vi "Optimize Function.vi"(3 "output control":T1, 4 "data":variant, 5 "X":dbl[](array[numeric])) -> (0 "error out":errorcluster, 1 "gradient":dbl[](array[numeric]), 2 "f(X)":dbl)   [LabVIEW 2016]
doc: "Use this template VI as a starting point to create an objective function you want to pass to the Unconstrained Optimization VI."
uses:
  <vilib>/Utility/error.llb/Error Cluster From Error Code.vi
  <vilib>/ErrorRing/Error Ring.xnode
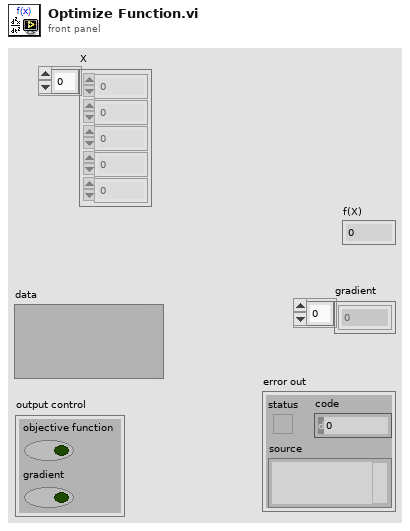
[diagram p1: front panel]
types:
  T1 = cluster{"objective function":bool, "gradient":bool}
  T2 = cluster{"c":dbl, "Intensity Graph":refnum<vi>, "animate?":bool}
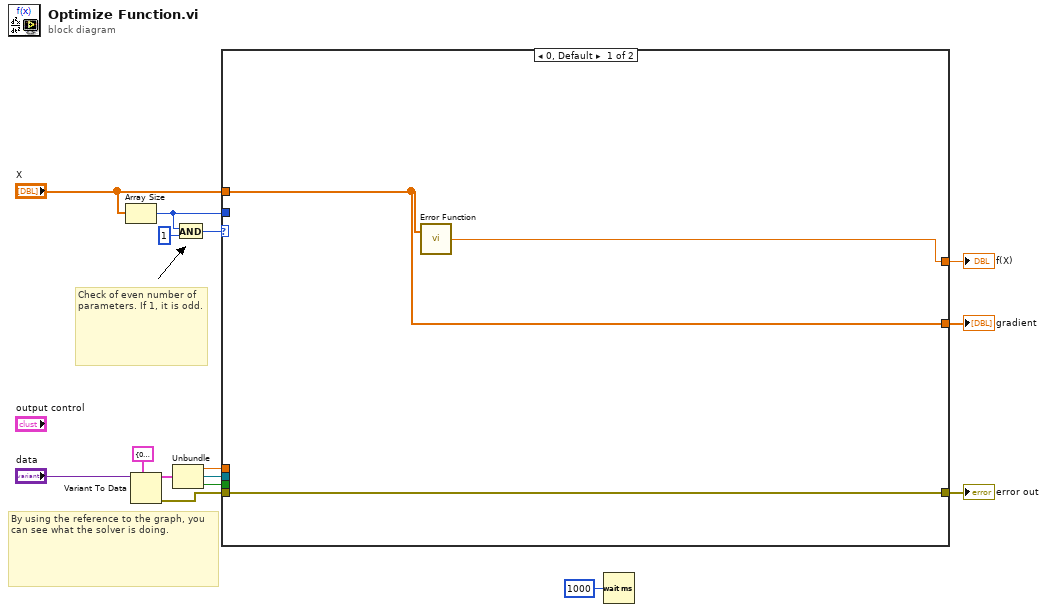
[diagram p0: block diagram]
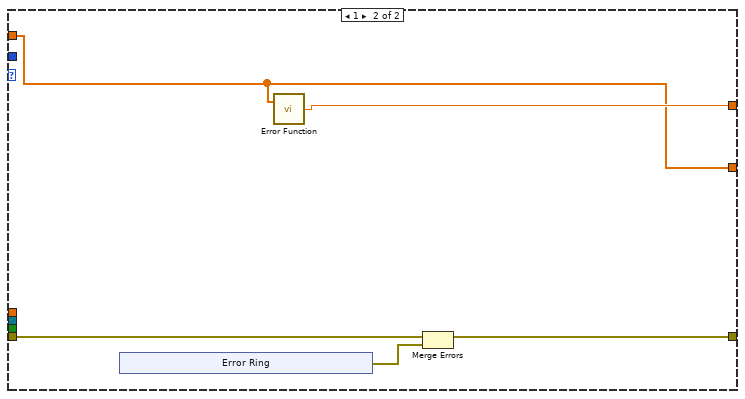
[diagram p2: hidden frame]
diagram:
  # "By using the reference to the graph, you can see what the solver is doing."
  # "Check of even number of parameters. If 1, it is odd."
  n1 = Array Size(array="X") -> (size(s)=w11:i32)
  n2 = Variant To Data(type=T2 {"c"=0.0, "Intensity Graph"=refnum, "animate?"=FALSE} ("output cluster"), Variant="data") -> (data=w9:T2, error out=w4:errorcluster)  [unwired: 1 in]
  n3 = Unbundle(w9) -> ("c"=w7:dbl, "Intensity Graph"=w6:refnum<vi>, "animate?"=w5:bool)
  n4 = And(x=w11, y=1) -> (x .and. y?=w14:i32)
  n5 = case shown="0, Default" w14 {
    tunnel: [w16 w22] -> w13
    tunnel: "X" -> [w17 w19]
    tunnel: w11 -> [_ _]
    tunnel: w7 -> [_ _]
    tunnel: w6 -> [_ _]
    tunnel: w5 -> [_ _]
    tunnel: w4 -> [w16 w23]
    tunnel: [w18 w20] -> w3
    tunnel: [w17 w19] -> w2
    frame 0, Default {
      n6 = call "Error Function.vi"("Array"=w17) -> ("Error"=w18:dbl)  [unwired: 1 in]
    }
    frame 1 {
      n7 = xnode "Error Ring"() -> ("error out"=w21:errorcluster)
      n8 = call "Error Function.vi"("Array"=w19) -> ("Error"=w20:dbl)  [unwired: 1 in]
      n9 = Merge Errors(w23, w21) -> (w22:errorcluster)
    }
  }
  "error out" <- w13
  "f(X)" <- w3
  "gradient" <- w2
  n10 = Wait (ms)(milliseconds to wait=u32 1000) -> ()  [unwired: 1 out]
